vi "Element Init.vi"(7 "VolatusAPI":refnum<class "VolatusAPI.lvclass">, 8 "error in (no error)":errorcluster, 10 "JSON":string, 11 "BluelinesRedlines in":refnum<class "BluelinesRedlines.lvclass">) -> (0 "error out":errorcluster, 3 "BluelinesRedlines out":refnum<class "BluelinesRedlines.lvclass">)   [LabVIEW 2020, in "VolatusGUIElements.lvlib" / "BluelinesRedlines.lvclass"]
uses:
  BluelinesRedlines.lvclass
  C:/dev/lv20CE/relink/lv-volatus/VolatusGUI/GUI Element/GUI Element.lvclass
  Volatus/VolatusAPI/VolatusAPI.lvclass
  VolatusGUI/GUI Element/GUI Element.lvclass/GUI Element.ctl
  BluelinesRedlines.lvclass/BluelinesRedlines.ctl
  VolatusGUI/GUI Element/GUI Element.lvclass
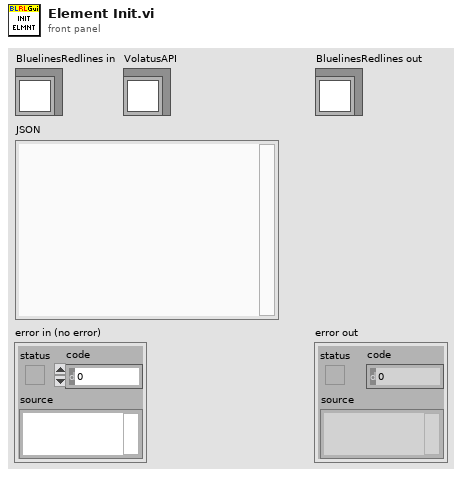
[diagram p1: front panel]
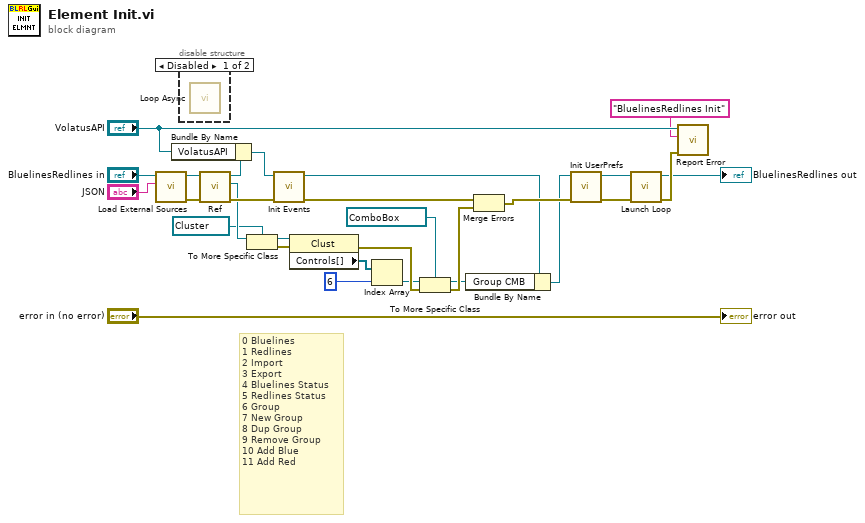
[diagram p0: block diagram]
diagram:
  # "0 Bluelines\n1 Redlines\n2 Import\n3 Export\n4 Bluelines Status\n5 Redlines Status\n6 Group\n7 New Group\n8 Dup Group\n9 Remove Group\n10 Add Blue\n11 Add Red"
  n1 = call "Load External Sources.vi"("JSON"="JSON", "BluelinesRedlines in"="BluelinesRedlines in") -> ("error out"=w19:errorcluster, "BluelinesRedlines out"=w22:refnum<class "BluelinesRedlines.lvclass">)  [unwired: 8 in]
  n2 = disable-structure shown="Disabled" {
    frame Disabled {
      n3 = call "Loop Async.vi"() -> ()  [unwired: 12 in]
    }
    frame Enabled {
    }
  }
  n4 = call "Ref.vi"("GUI Element in"=w22) -> ("Ref"=w11:refnum<vi>, "GUI Element out"=w12:refnum<class "BluelinesRedlines.lvclass">)  [unwired: 9 in]
  n5 = Bundle By Name(cluster=w12, "VolatusAPI"="VolatusAPI") -> (w15:refnum<class "BluelinesRedlines.lvclass">)
  n6 = To More Specific Class(target class=refnum<vi> refnum ("Group"), reference=w11) -> (specific class reference=w9:refnum<vi>, error out=w8:errorcluster)  [unwired: 1 in]
  n7 = call "Init Events.vi"("error in (no error)"=w19, "BluelinesRedlines in"=w15) -> ("error out"=w16:errorcluster, "BluelinesRedlines out"=w2:refnum<class "BluelinesRedlines.lvclass">)  [unwired: 8 in]
  n8 = property class="Clust"(reference=w9, error in=w8) -> (error out=w26:errorcluster, "Controls[]"=w7:refnum<vi>[])  [unwired: 1 out]
  n9 = Index Array(array=w7, index=6) -> (element=w5:refnum<vi>)
  n10 = To More Specific Class(target class=refnum<vi> refnum ("Group"), reference=w5, error in=w26) -> (specific class reference=w3:refnum<vi>, error out=w27:errorcluster)
  n11 = Bundle By Name(cluster=w2, "Group CMB"=w3) -> (w1:refnum<class "BluelinesRedlines.lvclass">)
  n12 = Merge Errors(w16, w27) -> (w28:errorcluster)
  n13 = call "Init UserPrefs.vi"("error in (no error)"=w28, "BluelinesRedlines in"=w1) -> ("error out"=w14:errorcluster, "BluelinesRedlines out"=w13:refnum<class "BluelinesRedlines.lvclass">)  [unwired: 8 in]
  n14 = call "Launch Loop.vi"("error in (no error)"=w14, "BluelinesRedlines in"=w13) -> ("error out"=w25:errorcluster, "BluelinesRedlines out"=→"BluelinesRedlines out":refnum<class "BluelinesRedlines.lvclass">)  [unwired: 8 in]
  n15 = call "Report Error.vi"("error in (no error)"=w25, "Context"="BluelinesRedlines Init", "VolatusAPI in"="VolatusAPI") -> ()  [unwired: 7 in, 2 out]
  "error out" <- "error in (no error)"
